vi "Shutdown.vi"(8 "error in (no error)":errorcluster, 11 "reference in":refnum<class "Test_Base.lvclass">) -> (0 "error out":errorcluster, 3 "reference in":refnum<class "Test_Base.lvclass">)   [LabVIEW 2022 SP3, in "Test_Base.lvlib" / "Test_Base.lvclass"]
uses:
  Test_Base.lvclass
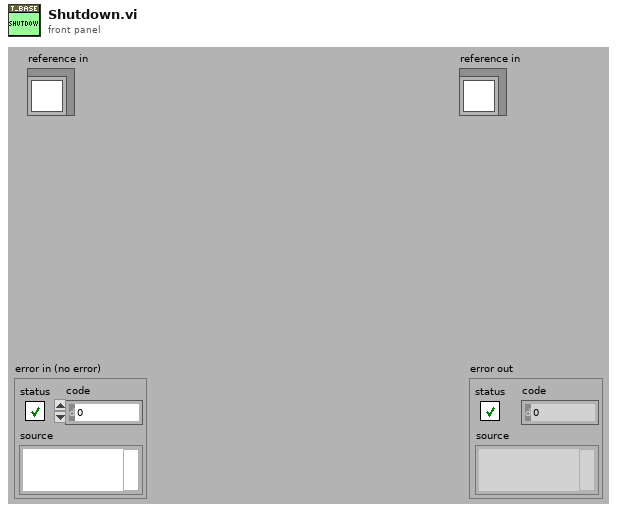
[diagram p1: front panel]
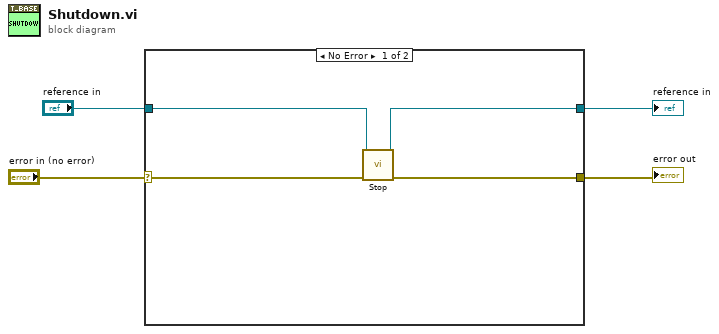
[diagram p0: block diagram]
diagram:
  n1 = case shown="No Error" "error in (no error)" {
    selector: "error in (no error)" -> [w6 w10]
    tunnel: [w5 w10] -> w3
    tunnel: [w7 w9] -> w1
    tunnel: "reference in" -> [w8 w9]
    frame No Error {
      n2 = call-dynamic "Stop.vi"("error in (no error)"=w6, "reference in"=w8) -> ("error out"=w5:errorcluster, "reference in"=w7:refnum<class "Test_Base.lvclass">)  [unwired: 8 in]
    }
    frame Error {
    }
  }
  "error out" <- w3
  "reference in" <- w1
